vi "Notify.vi"(8 "error in (no error)":errorcluster, 9 "ICallResult":refnum<class "ICallResult.lvclass">, 10 "Events":refnum<class "Events.lvclass">, 11 "CallRequest (JSON) in":refnum<class "CallRequest (JSON).lvclass">) -> (0 "error out":errorcluster, 3 "CallRequest (JSON) out":refnum<class "CallRequest (JSON).lvclass">)   [LabVIEW 2020, in "wamplv.lvlib" / "CallRequest (JSON).lvclass"]
uses:
  CallRequest (JSON).lvclass
  CallRequest (JSON).lvclass/CallRequest (JSON).ctl
  CallResult JSON/CallResult JSON.lvclass
  Events/EventsParent/Events.lvclass
  C:/local/wamplv/Private/Requests/Call/ICallResult/ICallResult.lvclass
  C:/local/wamplv/Private/Message loop classes/IRequestResult/IRequestResult.lvclass
  C:/local/wamplv/Private/Requests/Call/CallResult JSON/CallResult JSON.lvclass
  ICallResult/ICallResult.lvclass
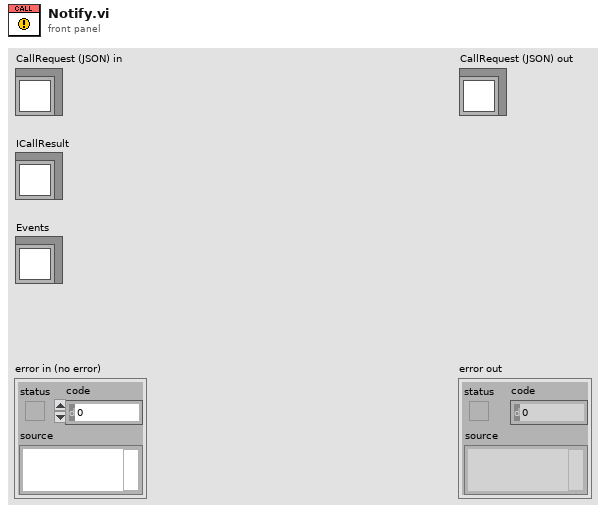
[diagram p1: front panel]
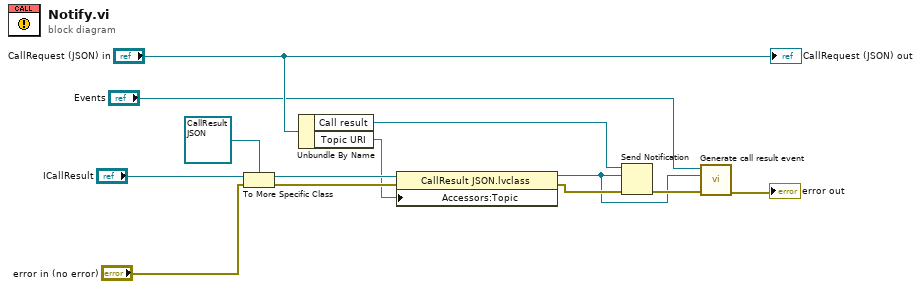
[diagram p0: block diagram]
diagram:
  n1 = To More Specific Class(target class=refnum<class "CallResult JSON.lvclass"> refnum ("wamplv.lvlib:CallResult JSON.lvclass"), reference="ICallResult", error in="error in (no error)") -> (specific class reference=w11:refnum<class "CallResult JSON.lvclass">, error out=w10:errorcluster)
  n2 = Unbundle By Name("CallRequest (JSON) in") -> ("Call result"=w4:refnum<notifier>, "Topic URI"=w8:string)
  n3 = property class="CallResult JSON.lvclass"(reference=w11, error in=w10, "Accessors:Topic"=w8) -> (reference out=w2:refnum<class "CallResult JSON.lvclass">, error out=w5:errorcluster)
  n4 = Send Notification(notification=w2, notifier=w4, error in (no error)=w5) -> (error out=w3:errorcluster)  [unwired: 1 out]
  n5 = call-dynamic "Generate call result event.vi"("error in (no error)"=w3, "ICallResult"=w2, "Events in"="Events") -> ("error out"=→"error out":errorcluster)  [unwired: 7 in, 1 out]
  "CallRequest (JSON) out" <- "CallRequest (JSON) in"
